vi "Write Map.vi"(8 "error in (no error)":errorcluster, 10 "Map":variant, 11 "JobReport in":refnum<class "JobReport.lvclass">) -> (0 "error out":errorcluster, 3 "JobReport out":refnum<class "JobReport.lvclass">)   [LabVIEW 2013, in "openCronJob.lvlib" / "JobReport.lvclass"]
uses:
  JobReport.lvclass
  JobReport.lvclass/JobReport.ctl
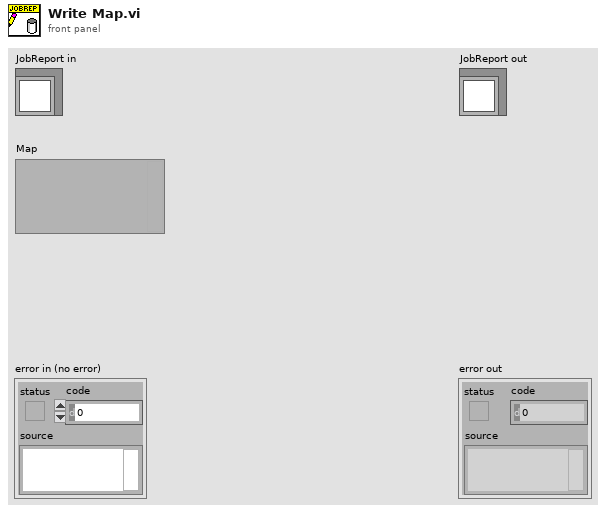
[diagram p1: front panel]
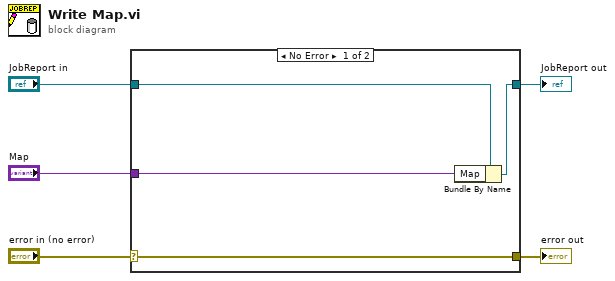
[diagram p0: block diagram]
diagram:
  n1 = case shown="No Error" "error in (no error)" {
    selector: "error in (no error)" -> [w9 w10]
    tunnel: [w9 w10] -> w4
    tunnel: [w7 w11] -> w2
    tunnel: "JobReport in" -> [w8 w11]
    tunnel: "Map" -> [w6 _]
    frame No Error {
      n2 = Bundle By Name(cluster=w8, "Map"=w6) -> (w7:refnum<class "JobReport.lvclass">)
    }
    frame Error {
    }
  }
  "error out" <- w4
  "JobReport out" <- w2
